vi "CounterSUBVI2.vi"() -> ()   [LabVIEW 2015]
panel:
  out "Numeric":i32
  out "x >= y?":bool
  in  "y":i32=15
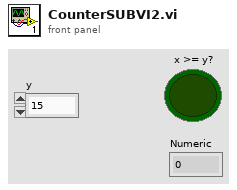
[diagram p1: front panel]
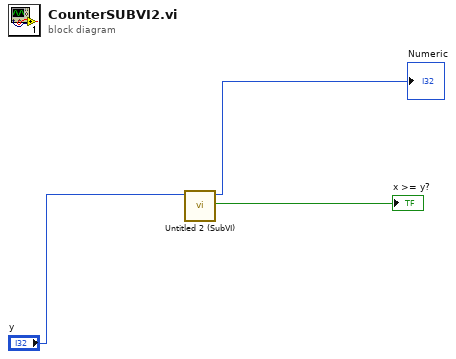
[diagram p0: block diagram]
diagram:
  n1 = call "Untitled 2 (SubVI).vi"("y"="y") -> ("Boolean"=→"x >= y?":bool, "Numeric"=→"Numeric":i32)  [unwired: 9 in]
